vi "WS1050 CAPDAC Setting.vi"(6 "DUT Mask Mode (All)":T1=enum."All", 8 "error in":errorcluster, 9 "C3 Cap DAC":u8=150 caption="B Data In" format="0x%02x", 10 "C2 Cap DAC":u8=134 caption="B Data In" format="0x%02x", 11 "C1 Cap DAC":u8=165 caption="B Data In" format="0x%02x") -> (0 "error out":errorcluster, 3 "AD7747 Values":string[][](table))   [LabVIEW 2012]
uses:
  WS_VCAP Driver 029/Source/WSVCAP Shell/Type Defs/WSVCAP SHL I2C DUT Mask Mode Enum.ctl
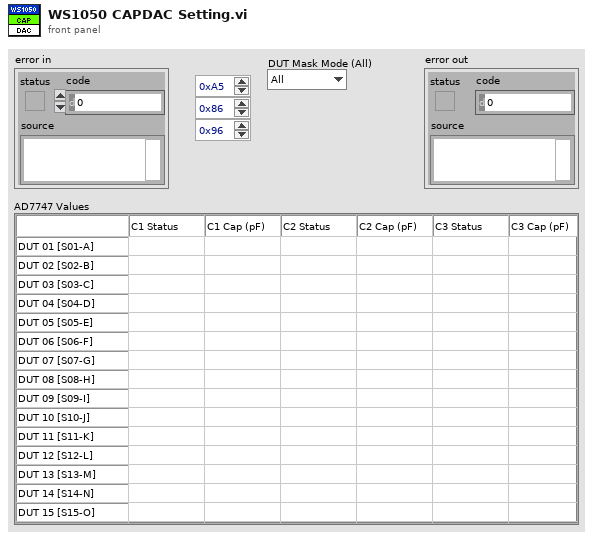
[diagram p1: front panel]
types:
  T1 = typedef "WSVCAP SHL I2C DUT Mask Mode Enum.ctl" = enum16{"Custom", "C1", "C2", "C3", "All"}
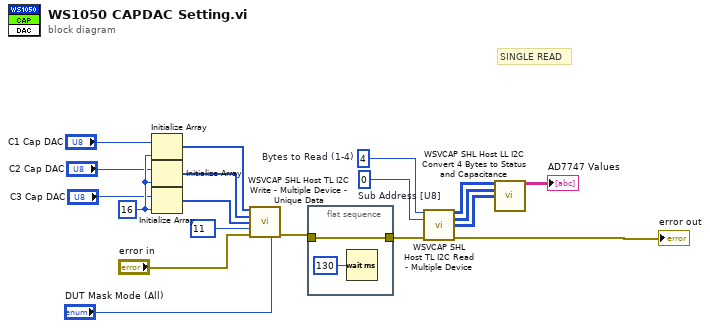
[diagram p0: block diagram]
diagram:
  w11 = 16 ("dimension size")
  w13 = u8 4  # Bytes to Read (1-4)
  w12 = u8 0  # Sub Address [U8]
  # "SINGLE READ"
  n1 = Initialize Array("C1 Cap DAC", w11) -> (w10:u8[])
  n2 = Initialize Array("C2 Cap DAC", w11) -> (w9:u8[])
  n3 = Initialize Array("C3 Cap DAC", w11) -> (w8:u8[])
  n4 = call "WSVCAP SHL Host TL I2C Write - Multiple Device - Unique Data.vi"("C1 Data"=w10, "C2 Data"=w9, "C3 Data"=w8, "Sub Address"=u8 11, "error in"="error in", "DUT Mask Mode (All)"="DUT Mask Mode (All)") -> ("error out"=w7:errorcluster)  [unwired: 9 in]
  n5 = flat-sequence {
    tunnel: w7 -> [w20]
    tunnel: [w20] -> w18
    frame #0 {
      n6 = Wait (ms)(milliseconds to wait=u32 130) -> ()  [unwired: 1 out]
    }
  }
  n7 = call "WSVCAP SHL Host TL I2C Read - Multiple Device.vi"("Bytes to Read (1-4)"=w13, "Sub Address [U8]"=w12, "error in"=w18) -> ("C1:1-36 Read Data [U8]"=w14:u8[][], "C2:1-36 Read Data [U8]"=w15:u8[][], "C3:1-36 Read Data [U8]"=w17:u8[][], "error out"=→"error out":errorcluster)  [unwired: 9 in]
  n8 = call "WSVCAP SHL Host LL I2C Convert 4 Bytes to Status and Capacitance.vi"("C1:1-36 Read Data [U8]"=w14, "C2_1-36 Read Data [U8]"=w15, "C3_1-36 Read Data [U8]"=w17) -> ("AD7747 Values"=→"AD7747 Values":string[][])  [unwired: 12 in]
